vi "Create New Filled Text Fields.vi"(8 "error in (no error)":errorcluster, 11 "Filled Text Fields Ref":refnum<vi>) -> (0 "error out":errorcluster, 3 "Filled Text Fields out":refnum<class "Filled Text Fields.lvclass">)   [LabVIEW 2017, in "Filled Text Fields Actor.lvlib" / "Filled Text Fields.lvclass"]
uses:
  Filled Text Fields.lvclass
  Filled Text Fields.lvclass/Filled Text Fields.ctl
  Filled Text Fields Actor/Filled Text Fields Actor.lvclass
  Filled Text Fields Actor Messages/Get SyncData Msg/Get SyncData Msg.lvclass
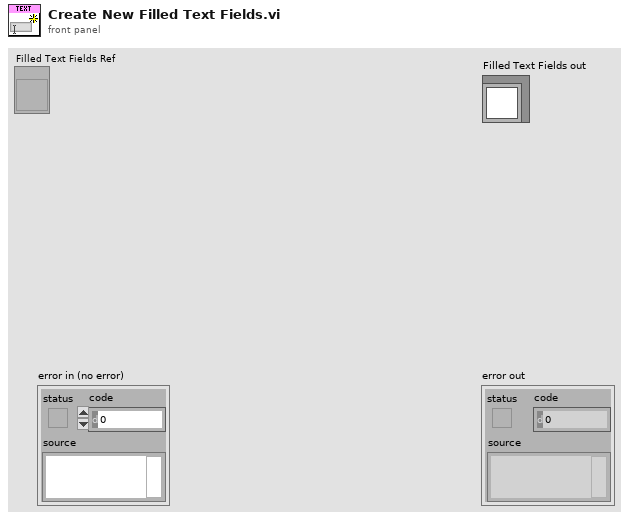
[diagram p1: front panel]
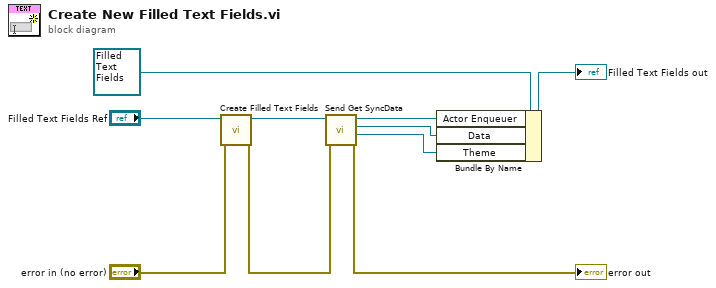
[diagram p0: block diagram]
diagram:
  n1 = call "Create Filled Text Fields.vi"("error in (no error)"="error in (no error)", "Filled Text Fields Ref"="Filled Text Fields Ref") -> ("error out"=w2:errorcluster, "Filled Text Fields Reference"=w6:refnum<class "Message Enqueuer.lvclass">)  [unwired: 8 in]
  n2 = call "Send Get SyncData.vi"("error in (no error)"=w2, "Message Enqueuer in"=w6) -> ("error out"=→"error out":errorcluster, "Theme"=w3:refnum<class "Theme.lvclass">, "Data"=w4:refnum<class "Data.lvclass">, "Message Enqueuer out"=w5:refnum<class "Message Enqueuer.lvclass">)  [unwired: 6 in]
  n3 = Bundle By Name(cluster=refnum<class "Filled Text Fields.lvclass"> refnum ("Filled Text Fields in"), "Actor Enqueuer"=w5, "Data"=w4, "Theme"=w3) -> (→"Filled Text Fields out":refnum<class "Filled Text Fields.lvclass">)
